vi "Vertical Profile.vi"(6 "Averaging time (min)":dbl, 7 "Lat.Coords":T1={"X"=-3390.0, "Y"=-113.0, "Z"=780.0, "Name"="Anemo1", "Spacing"=enum."Specified", "start"=780.0, "end"=780.0, "NumPts"=780.0, "Specified Locns"=[]}, 9 "Direction":enum16{"Forward", "Reverse"}(ring), 10 "Tunnel Speed":dbl, 11 "Input Task Array":T2[](array[typedef]) {"Carrier_2 Q (l/min)" format="%#.2f"; "Row Duration (mins)" format="%#.1f"; "Row No" min=0; "Trace Gas Concentration (%)" min=0.0 format="%#_4f"; "Carrier_1 Q (l/min)" format="%#.2f"; "Tunnel Speed" format="%#.2f"; "Start X" format="%#.2f"; "Start Y" format="%#.2f"; "Start Z" format="%#.2f"; "End X" format="%#.2f"; "End Y" format="%#.2f"; "End Z" format="%#.2f"; "Averaging time (min)" min=0.0 format="%#.2f"}) -> (3 "Output Task Array":T2[](array[typedef]) {"Carrier_2 Q (l/min)" format="%#.2f"; "Row Duration (mins)" format="%#.1f"; "Row No" min=0; "Trace Gas Concentration (%)" min=0.0 format="%#_4f"; "Carrier_1 Q (l/min)" format="%#.2f"; "Tunnel Speed" format="%#.2f"; "Start X" format="%#.2f"; "Start Y" format="%#.2f"; "Start Z" format="%#.2f"; "End X" format="%#.2f"; "End Y" format="%#.2f"; "End Z" format="%#.2f"; "Averaging time (min)" min=0.0 format="%#.2f"})   [LabVIEW 2022 SP3]
uses:
  RowTemplate.ctl
  Anemometry Sub Vis/Gen Trav/Spacing.ctl
  Anemometry Sub Vis/Controls/Multi_run_mode.ctl
  <vilib>/Analysis/baseanly.llb/Mean (DBL).vi
  MRCMDFBGlobal.vi
  Set ADAM Ch.vi
  <vilib>/Analysis/NI_AALBase.lvlib
panel:
  out "dz":dbl
  # "X           Y            Z"
  # "Start"
  # "End"
  # "X           Y            Z"
  # "Start"
  # "End"
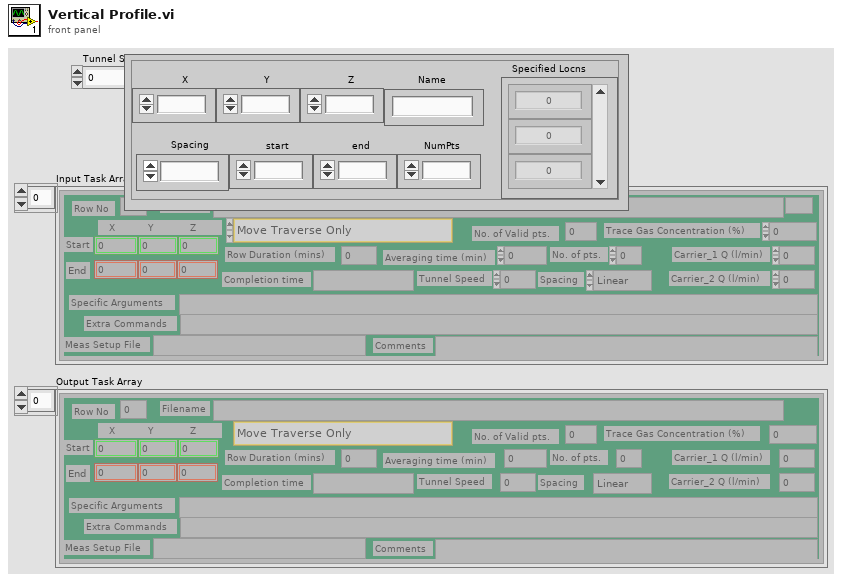
[diagram p1: front panel]
types:
  T1 = cluster{"X":dbl, "Y":dbl, "Z":dbl, "Name":string, "Spacing":enum16{"Linear", "Log", "Gauss", "Specified", "N/A"}, "start":dbl, "end":dbl, "NumPts":dbl, "Specified Locns":dbl[]}
  T2 = typedef "RowTemplate.ctl" = cluster{"Start X":sgl, "Start Y":sgl, "Start Z":sgl, "End X":sgl, "End Y":sgl, "End Z":sgl, "No. of pts.":i32, "Spacing":T3, "Filename":path, "Tunnel Speed":dbl, "Averaging time (min)":dbl, "Extra Commands":string, "Carrier_1 Q (l/min)":dbl, "Carrier_2 Q (l/min)":dbl, "Trace Gas Concentration (%)":dbl, "Specific Arguments":string, "Comments":string, "Row No":i32, "Row Type Selector":T4, "Completion time":string, "Row Duration (mins)":dbl, "No. of Valid pts.":i32, "Meas Setup File":string}
  T3 = typedef "Spacing.ctl" = enum16{"Linear", "Log", "Gauss", "Specified", "N/A"}
  T4 = typedef "Multi_run_mode.ctl" = enum16{"Move Traverse Only", "Set Tunnel Speed Only", "Set Source Only", "Set Measurement Conditions", "Single Measurement", "Vertical Profile", "Lateral Profile", "Longitudinal Profile", "Multi-Axis Profile", "Explore Volume", "Auto Calibrate", "Meas Fast FID Bkgnd", "Check Beam Power", "Scanning Valve Measurement", "Run VI Named:", "Set ADAM Ch", "Wait (minutes)", "Send Message", "Synchronize With:", "Fall Back to this Row", "Turn Off Row Repeating", "Traverse 3D Volume", "Blank Row", "Jump to Fall Back Row"}
  T5 = cluster{"Start X":sgl, "Start Y":sgl, "Start Z":sgl, "End X":sgl, "End Y":sgl, "End Z":sgl, "No. of pts.":i32, "Spacing":T3, "Filename":path, "Tunnel Speed":dbl, "Averaging time (min)":dbl, "Extra Commands":string, "Carrier_1 Q (l/min)":dbl, "Carrier_2 Q (l/min)":dbl, "Trace Gas Concentration (%)":dbl, "Specific Arguments":string, "Comments":string, "Row No":i32, "Row Type Selector":T4, "Completion time":string, "Row Duration (mins)":dbl, "No. of Valid pts.":i32, "Meas Setup File":string}[]
  T6 = cluster{"Start X":sgl, "Start Y":sgl, "Start Z":sgl, "End X":sgl, "End Y":sgl, "End Z":sgl, "No. of pts.":i32, "Spacing":T3, "Filename":path, "Tunnel Speed":dbl, "Averaging time (min)":dbl, "Extra Commands":string, "Carrier_1 Q (l/min)":dbl, "Carrier_2 Q (l/min)":dbl, "Trace Gas Concentration (%)":dbl, "Specific Arguments":string, "Comments":string, "Row No":i32, "Row Type Selector":T4, "Completion time":string, "Row Duration (mins)":dbl, "No. of Valid pts.":i32, "Meas Setup File":string}
  T7 = typedef "CorrectionsCluster.ctl" = cluster{"Use Height Corrections":bool, "TT.Azimuths":dbl[], "Z.HeightCorrs":dbl[][], "Corrections from File":bool, "Height Survey Filepaths":path[]}
  T8 = cluster{"Azimuth Array Index":u32, "Vert Prof Array Index":u32, "Lat Prof Array Index":u32, "Long Prof Array Index":u32}
  T9 = typedef "ProfCoords.ctl" = cluster{"X":dbl, "Y":dbl, "Z":dbl, "Name":string, "Spacing":enum16{"Linear", "Log", "Gauss", "Specified", "N/A"}, "start":dbl, "end":dbl, "NumPts":dbl, "Specified Locns":dbl[]}[]
  T10 = enum16{"Linear", "Log", "Gauss", "Specified", "N/A"}
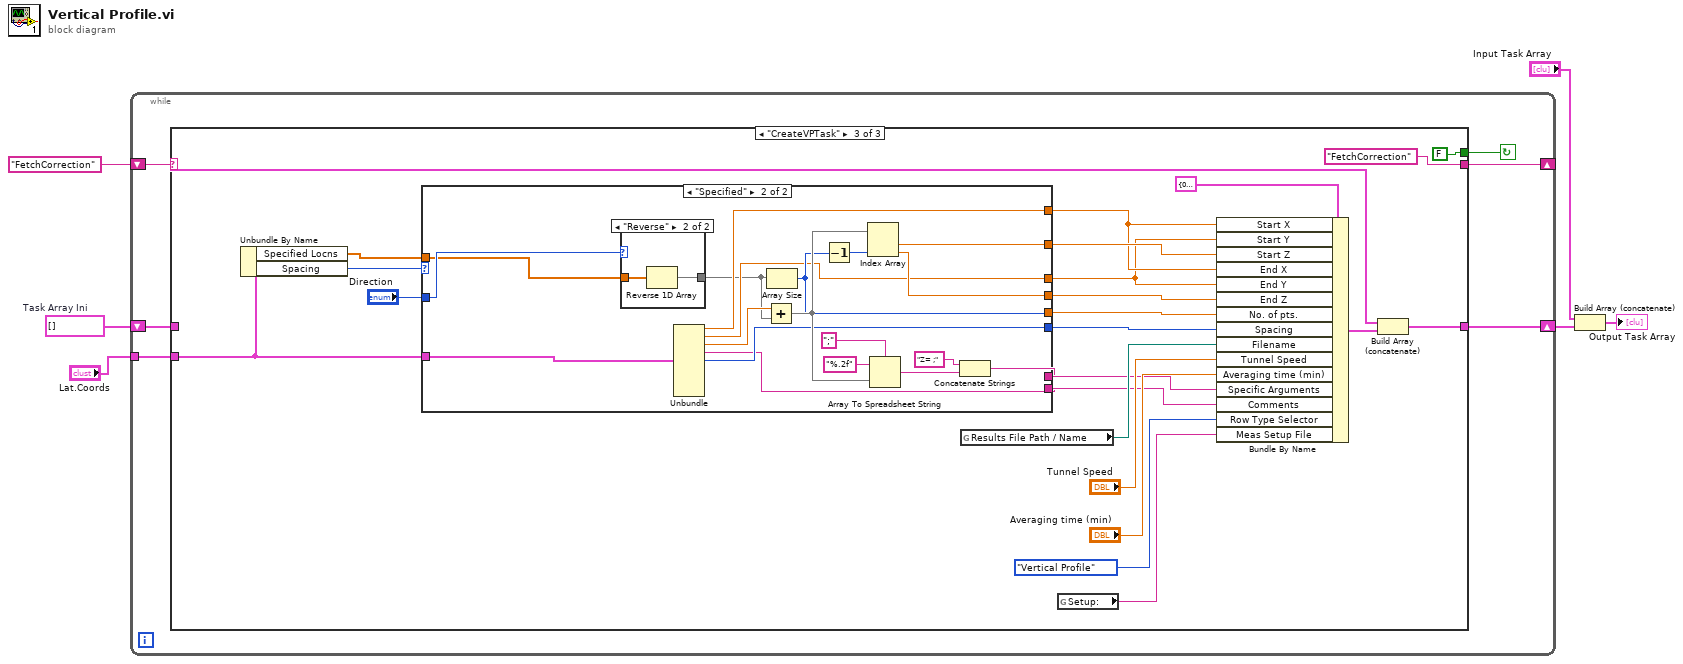
[diagram p0: block diagram]
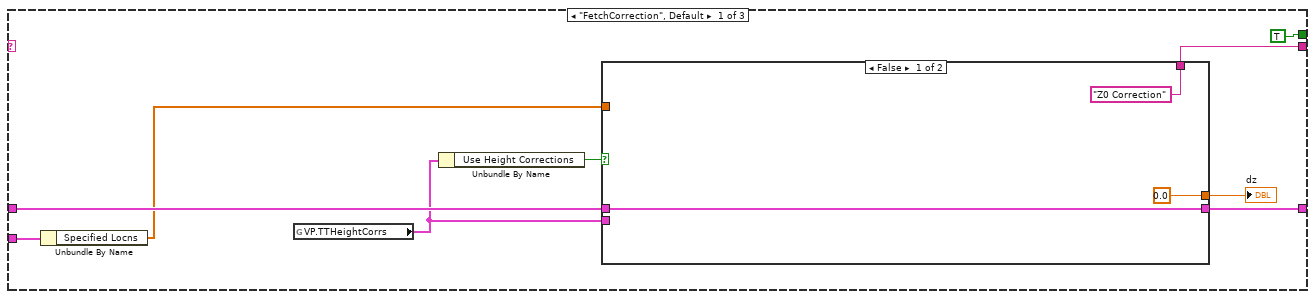
[diagram p2: hidden frame]
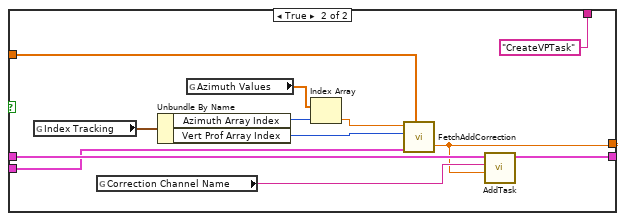
[diagram p3: hidden frame]
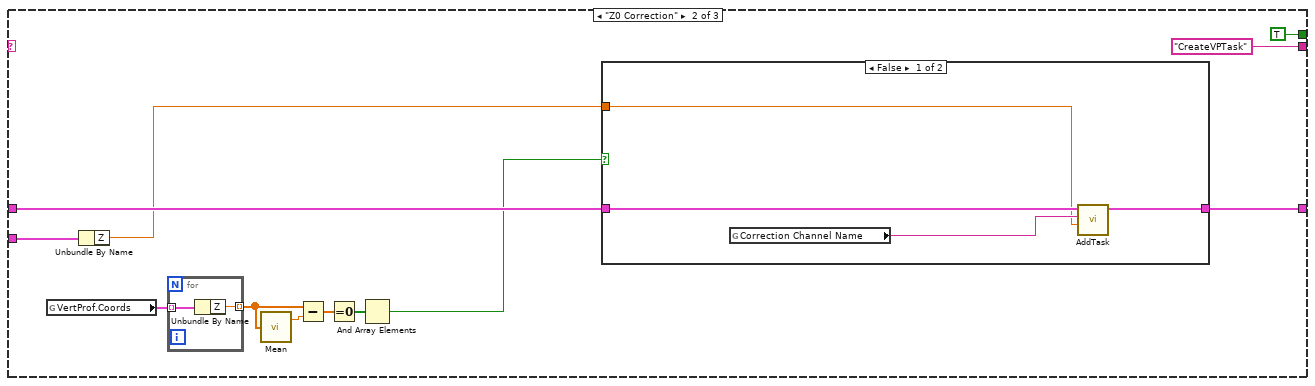
[diagram p4: hidden frame]
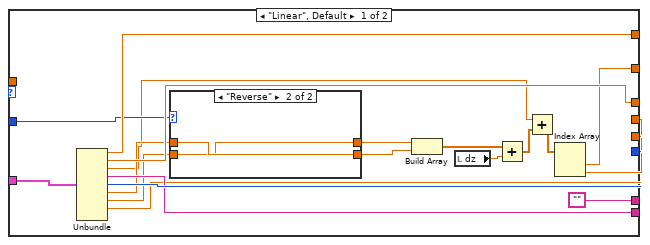
[diagram p6: hidden frame]
diagram:
  w2 = T5 []  # Task Array Ini
  n1 = while {
    shift-right: [w8] -> _
    shift-left: "FetchCorrection" -> [w11]
    shift-right: [w12] -> w4
    shift-left: w2 -> [w10]
    tunnel: "Lat.Coords" -> [w7]
    stop <- w9 continue-if-true
    n2 = case shown="\"CreateVPTask\"" w11 {
      tunnel: [w20 w47 w66] -> w12
      tunnel: [w13 "CreateVPTask" "FetchCorrection"] -> w8
      tunnel: w10 -> [w21 w48 w65]
      tunnel: [TRUE TRUE FALSE] -> w9
      tunnel: w7 -> [w15 w45 w56]
      frame "FetchCorrection", Default {
        n3 = Unbundle By Name(w15) -> ("Specified Locns"=w14:dbl[])
        n4 = global read "MRCMDFBGlobal.vi" "VP.TTHeightCorrs"() -> (w18:T7)
        n5 = Unbundle By Name(w18) -> ("Use Height Corrections"=w17:bool)
        n6 = case shown="False" w17 {
          tunnel: w21 -> [w24 w33]
          tunnel: [w24 w32] -> w20
          tunnel: w18 -> [_ w28]
          tunnel: [0.0 ("dz") w27] -> w16
          tunnel: w14 -> [_ w26]
          tunnel: ["Z0 Correction" "CreateVPTask"] -> w13
          frame False {
          }
          frame True {
            n7 = global read "MRCMDFBGlobal.vi" "Index Tracking"() -> (w36:T8)
            n8 = global read "MRCMDFBGlobal.vi" "Correction Channel Name"() -> (w34:string)
            n9 = Unbundle By Name(w36) -> ("Azimuth Array Index"=w30:u32, "Vert Prof Array Index"=w35:u32)
            n10 = global read "MRCMDFBGlobal.vi" "Azimuth Values"() -> (w31:dbl[])
            n11 = Index Array(array=w31, index=w30) -> (element=w29:dbl)
            n12 = call "FetchAddCorrection.vi"("Azimuth Value"=w29, "Vert Prof Array Index"=w35, "VP.TTHeightCorrs"=w28, "Vert.Z-Locations"=w26) -> ("dz"=w27:dbl)  [unwired: 1 in, 1 out]
            n13 = call-poly "AddTask.vi"("Value"=w27, "ADAM:Channel:Name"=w34, "Input Task Array"=w33) -> ("Output Task Array"=w32:T2[])  [unwired: 8 in]
          }
        }
        "dz" <- w16
      }
      frame "Z0 Correction" {
        n14 = global read "MRCMDFBGlobal.vi" "VertProf.Coords"() -> (w43:T9)
        n15 = Unbundle By Name(w45) -> ("Z"=w44:dbl)
        n16 = for {
          tunnel: w43 -> [w50] mode=indexing
          tunnel: [w49] -> w41 mode=indexing
          n17 = Unbundle By Name(w50) -> ("Z"=w49:dbl)
        }
        n18 = call-poly <vilib>:"Mean.vi"("X"=w41) -> ("mean"=w42:dbl)  [unwired: 1 out]
        n19 = Subtract(x=w41, y=w42) -> (x-y=w40:dbl[])
        n20 = Equal To 0?(x=w40) -> (x = 0?=w39:bool[])
        n21 = And Array Elements(Boolean array=w39) -> (logical AND=w38:bool)
        n22 = case shown="False" w38 {
          tunnel: w48 -> [w53 w55]
          tunnel: [w52 w55] -> w47
          tunnel: w44 -> [w51 _]
          frame False {
            n23 = global read "MRCMDFBGlobal.vi" "Correction Channel Name"() -> (w54:string)
            n24 = call-poly "AddTask.vi"("Value"=w51, "ADAM:Channel:Name"=w54, "Input Task Array"=w53) -> ("Output Task Array"=w52:T2[])  [unwired: 8 in]
          }
          frame True {
          }
        }
      }
      frame "CreateVPTask" {
        n25 = Unbundle By Name(w56) -> ("Specified Locns"=w57:dbl[], "Spacing"=w63:T10)
        n26 = case shown="\"Specified\"" w63 {
          tunnel: ["" w114] -> w72
          tunnel: [w92 w113] -> w71
          tunnel: [w88 w112] -> w70
          tunnel: [w87 w111] -> w69
          tunnel: w56 -> [w97 w110]
          tunnel: [w96 w106] -> w62
          tunnel: [w95 w105] -> w61
          tunnel: [w94 w109] -> w60
          tunnel: [w93 w108] -> w59
          tunnel: "Direction" -> [w86 w104]
          tunnel: w57 -> [_ w102]
          frame "Linear", Default {
            n27 = Unbundle(w97) -> ("X"=w94:dbl, "Y"=w93:dbl, "Z"=w80:dbl, "Name"=w95:string, "Spacing"=w96:T10, "start"=w85:dbl, "end"=w83:dbl, "NumPts"=w92:dbl)  [unwired: 1 out]
            n28 = case shown="\"Reverse\"" w86 {
              tunnel: w85 -> [w99 w101]
              tunnel: [w99 w100] -> w84
              tunnel: w83 -> [w98 w100]
              tunnel: [w98 w101] -> w82
              frame "Forward", Default {
              }
              frame "Reverse" {
              }
            }
            n29 = Build Array(w84, w82) -> (w89:dbl[])
            n30 = local read "dz"() -> (w90:dbl)
            n31 = Add(x=w89, y=w90) -> (x+y=w81:dbl[])
            n32 = Add(x=w80, y=w81) -> (x+y=w79:dbl[])
            n33 = Index Array(array=w79) -> (element #1=w88:dbl, element #2=w87:dbl)  [unwired: 2 in]
          }
          frame "Specified" {
            n34 = case shown="\"Reverse\"" w104 {
              tunnel: [w121 w122] -> w103
              tunnel: w102 -> [w121 w123]
              frame "Forward", Default {
              }
              frame "Reverse" {
                n35 = Reverse 1D Array(array=w123) -> (reversed array=w122:dbl[])
              }
            }
            n36 = Unbundle(w110) -> ("X"=w109:dbl, "Y"=w108:dbl, "Z"=w107:dbl, "Name"=w105:string, "Spacing"=w106:T10)  [unwired: 4 out]
            n37 = Add(x=w107, y=w103) -> (x+y=w120:dbl[])
            n38 = Array Size(array=w103) -> (size(s)=w113:i32)
            n39 = Decrement(x=w113) -> (x-1=w117:i32)
            n40 = Index Array(array=w120, index #2=w117) -> (element #1=w112:dbl, element #2=w111:dbl)  [unwired: 1 in]
            n41 = Array To Spreadsheet String(delimiter (Tab)=";", array=w120, 3:"%.2f" ("format string")) -> (spreadsheet string=w118:string)
            n42 = Concatenate Strings("Z= ;", w118) -> (w114:string)
          }
        }
        n43 = global read "MRCMDFBGlobal.vi" "Results File Path / Name"() -> (w73:path)
        n44 = global read "MRCMDFBGlobal.vi" "Setup:"() -> (w74:string)
        n45 = Bundle By Name(cluster=T6 {"Start X"=0.0, "Start Y"=0.0, "Start Z"=0.0, "End X"=0.0, "End Y"=0.0, "End Z"=0.0, "No. of pts."=0, "Spacing"=enum."Linear", "Filename"=path "", "Tunnel Speed"=0.0, "Averaging time (min)"=0.0, "Extra Commands"="", "Carrier_1 Q (l/min)"=0.0, "Carrier_2 Q (l/min)"=0.0, "Trace Gas Concentration (%)"=0.0, "Specific Arguments"="", "Comments"="", "Row No"=0, "Row Type Selector"=enum."Move Traverse Only", "Completion time"="", "Row Duration (mins)"=0.0, "No. of Valid pts."=0, "Meas Setup File"=""} ("RowTemplateConst"), "Start X"=w60, "Start Y"=w59, "Start Z"=w70, "End X"=w60, "End Y"=w59, "End Z"=w69, "No. of pts."=w71, "Spacing"=w62, "Filename"=w73, "Tunnel Speed"="Tunnel Speed", "Averaging time (min)"="Averaging time (min)", "Specific Arguments"=w72, "Comments"=w61, "Row Type Selector"=Multi_run_mode."Vertical Profile", "Meas Setup File"=w74) -> (w67:T6)
        n46 = Build Array (concatenate)(w65, w67) -> (w66:T2[])
      }
    }
  }
  n47 = Build Array (concatenate)("Input Task Array", w4) -> (→"Output Task Array":T2[])
